vi "Set QueryResponse.vi"(7 "Complete Call (T)":bool=TRUE, 8 "error in (no error)":errorcluster, 10 "QueryResponse_Data":T1, 11 "gRPCid":T2) -> (0 "error out":errorcluster)   [LabVIEW 2019, in "OOP Server.lvlib" / "OOP Server.lvclass"]
uses:
  OOP Server.lvclass
  gRPC interface/Server API/typeDefs/grpcId.ctl
  QueryResponse_Data.ctl
  a54c73d7-c73e-42e8-801b-f6c5b1689305.vi
  <vilib>/Utility/error.llb/Error Cluster From Error Code.vi
  gRPC interface/gprc-lvsupport.lvlib
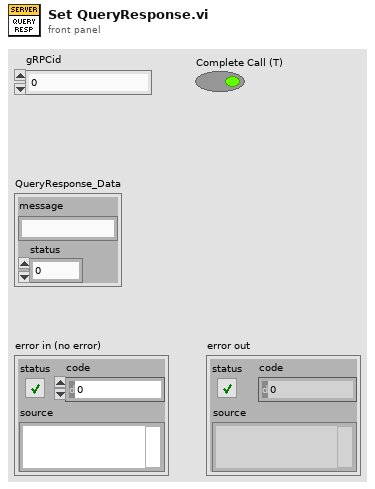
[diagram p1: front panel]
types:
  T1 = typedef "OOP Server.lvlib/OOP Server.lvclass/QueryResponse_Data.ctl" = cluster{"message":string, "status":i32}
  T2 = typedef "gprc-lvsupport.lvlib/grpcId.ctl" = u64
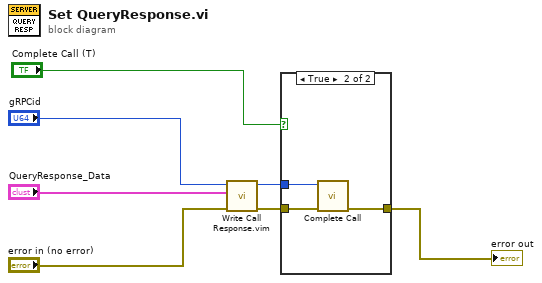
[diagram p0: block diagram]
diagram:
  n1 = call "Write Call Response.vim"("error in (no error)"="error in (no error)", "Response Data"="QueryResponse_Data", "gRPCid in"="gRPCid") -> ("error out"=w6:errorcluster, "gRPCid"=w5:T2)  [unwired: 7 in]
  n2 = case shown="True" "Complete Call (T)" {
    tunnel: [w8 w11] -> w7
    tunnel: w6 -> [w8 w10]
    tunnel: w5 -> [_ w9]
    frame False {
    }
    frame True {
      n3 = call "Complete Call.vi"("gRPCid"=w9, "error in (no error)"=w10) -> ("error out"=w11:errorcluster)  [unwired: 8 in]
    }
  }
  "error out" <- w7
